vi "Read and Write Visa.vi"(8 "error in (no error)":errorcluster, 10 "Command to Send":string, 11 "VISA Refnum in":refnum<visa-resource-name>) -> (0 "error out":errorcluster, 2 "Expected Response out":string, 3 "VISA Refnum out":refnum<visa-resource-name>)   [LabVIEW 2020, in "UI Actor.lvlib" / "UI Actor.lvclass"]
uses:
  UI Actor.lvclass
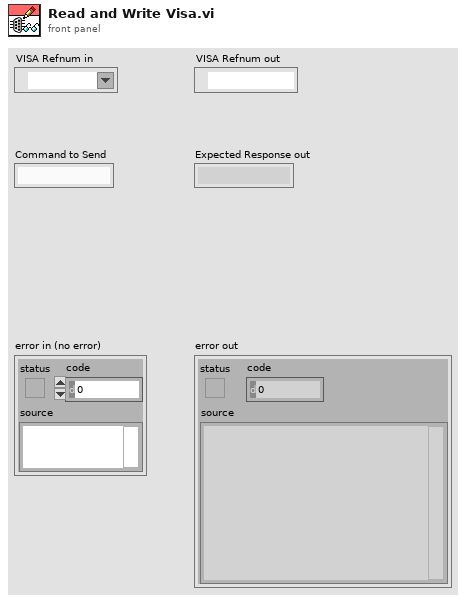
[diagram p1: front panel]
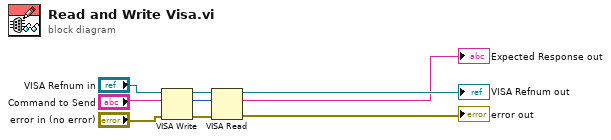
[diagram p0: block diagram]
diagram:
  n1 = VISA Write(VISA resource name="VISA Refnum in", write buffer="Command to Send", error in (no error)="error in (no error)") -> (VISA resource name out=w4:refnum<visa-resource-name>, return count=w2:u32, error out=w3:errorcluster)
  n2 = VISA Read(VISA resource name=w4, byte count=w2, error in (no error)=w3) -> (VISA resource name out=→"VISA Refnum out":refnum<visa-resource-name>, read buffer=→"Expected Response out":string, error out=→"error out":errorcluster)  [unwired: 1 out]
